vi "更新列首行首.vi"(0 "MulticolumnListbox输入":refnum<vi>, 1 "Coords":T1, 3 "列首？":bool=TRUE, 4 "行首？":bool=TRUE, 5 "项名？":bool=TRUE, 7 "编辑单元格":bool=TRUE) -> (13 "边界内？":bool, 14 "列首":string[](array[string]), 16 "行首":string[](array[string]), 18 "项名":string[][](array[string]), 19 "错误输出":errorcluster)   [LabVIEW 2016]
uses:
  <vilib>/Utility/miscctls.llb/LVPoint32TypeDef.ctl
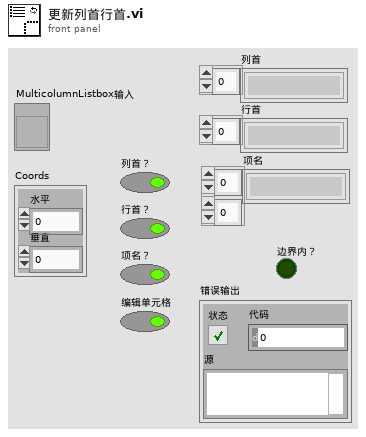
[diagram p1: front panel]
types:
  T1 = typedef "LVPoint32TypeDef.ctl" = cluster{"Horizontal":i32, "Vertical":i32}
  T2 = typedef "LVRowAndColumnTypeDef.ctl" = cluster{"Row":i32, "Column":i32}
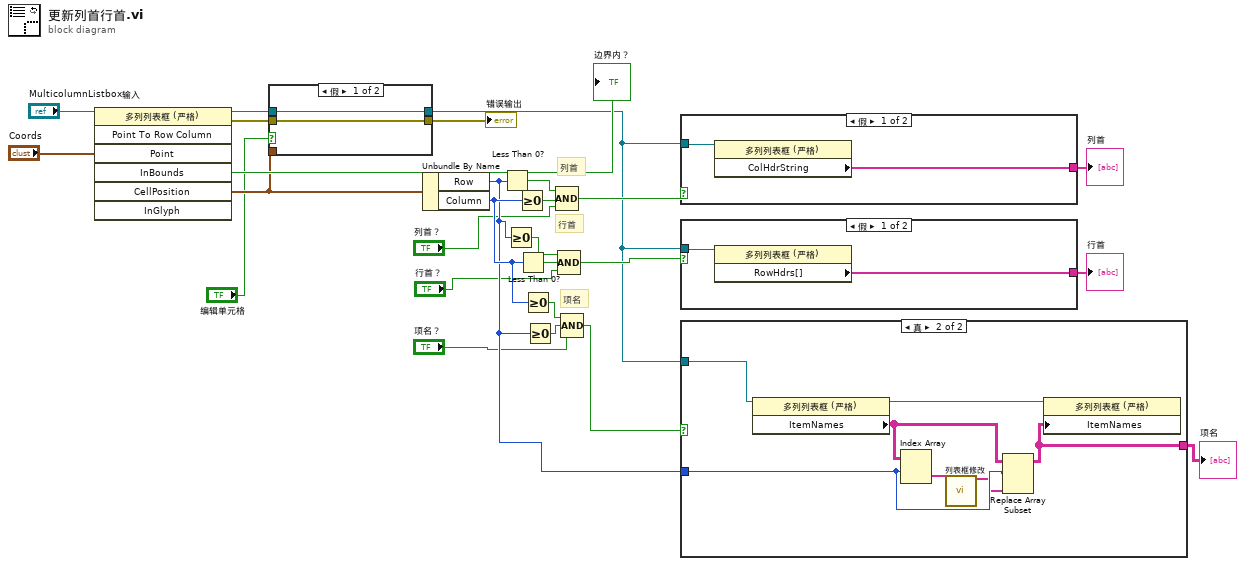
[diagram p0: block diagram]
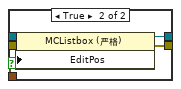
[diagram p2: hidden frame]
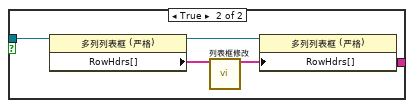
[diagram p3: hidden frame]
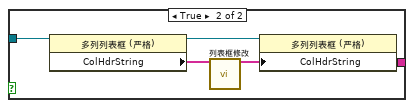
[diagram p4: hidden frame]
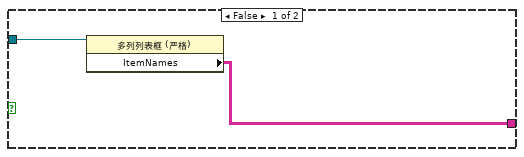
[diagram p5: hidden frame]
diagram:
  # "项名"
  # "列首"
  # "行首"
  n1 = invoke class="多列列表框 (严格)" method="Point To Row Column"(reference="MulticolumnListbox输入", "Point"="Coords") -> (reference out=w6:refnum<vi>, error out=w4:errorcluster, "InBounds"=→"边界内？":bool, "CellPosition"=w2:T2)  [unwired: 5 in, 3 out]
  n2 = case shown="假" "编辑单元格" {
    tunnel: w6 -> [w28 w33]
    tunnel: [w28 w32] -> w5
    tunnel: w4 -> [w27 w31]
    tunnel: [w27 w30] -> w3
    tunnel: w2 -> [_ w29]
    frame False {
    }
    frame True {
      n3 = property class="MCListbox (严格)"(reference=w33, error in=w31, "EditPos"=w29) -> (reference out=w32:refnum<vi>, error out=w30:errorcluster)
    }
  }
  "错误输出" <- w3
  n4 = Unbundle By Name(w2) -> ("Row"=w13:i32, "Column"=w14:i32)
  n5 = Less Than 0?(x=w13) -> (x < 0?=w23:bool)
  n6 = Greater Or Equal To 0?(x=w13) -> (x >= 0?=w22:bool)
  n7 = Greater Or Equal To 0?(x=w14) -> (x >= 0?=w24:bool)
  n8 = Less Than 0?(x=w14) -> (x < 0?=w21:bool)
  n9 = Greater Or Equal To 0?(x=w14) -> (x >= 0?=w12:bool)
  n10 = Greater Or Equal To 0?(x=w13) -> (x >= 0?=w11:bool)
  n11 = Compound Arithmetic op=AND ("复合运算")(w23, w24, "列首？") -> (w19:bool)
  n12 = Compound Arithmetic op=AND ("复合运算")(w22, w21, "行首？") -> (w18:bool)
  n13 = Compound Arithmetic op=AND ("复合运算")(w12, w11, "项名？") -> (w10:bool)
  n14 = case shown="假" w19 {
    tunnel: w5 -> [w35 w37]
    tunnel: [w34 w36] -> w17
    frame False {
      n15 = property class="多列列表框 (严格)"(reference=w35) -> ("ColHdrString"=w34:string[])  [unwired: 1 in, 2 out]
    }
    frame True {
      n16 = property class="多列列表框 (严格)"(reference=w37) -> (reference out=w38:refnum<vi>, "ColHdrString"=w39:string[])  [unwired: 1 in, 1 out]
      n17 = call "列表框修改.vi"("输入/修改"=w39) -> ("增加测试信息"=w36:string[])  [unwired: 13 in, 1 out]
      n18 = property class="多列列表框 (严格)"(reference=w38, "ColHdrString"=w36) -> ()  [unwired: 1 in, 2 out]
    }
  }
  "列首" <- w17
  n19 = case shown="假" w18 {
    tunnel: w5 -> [w41 w43]
    tunnel: [w40 w42] -> w16
    frame False {
      n20 = property class="多列列表框 (严格)"(reference=w41) -> ("RowHdrs[]"=w40:string[])  [unwired: 1 in, 2 out]
    }
    frame True {
      n21 = property class="多列列表框 (严格)"(reference=w43) -> (reference out=w44:refnum<vi>, "RowHdrs[]"=w45:string[])  [unwired: 1 in, 1 out]
      n22 = call "列表框修改.vi"("输入/修改"=w45) -> ("增加测试信息"=w42:string[])  [unwired: 13 in, 1 out]
      n23 = property class="多列列表框 (严格)"(reference=w44, "RowHdrs[]"=w42) -> ()  [unwired: 1 in, 2 out]
    }
  }
  "行首" <- w16
  n24 = case shown="真" w10 {
    tunnel: w13 -> [_ w51]
    tunnel: w5 -> [w47 w53]
    tunnel: [w46 w48] -> w15
    frame False {
      n25 = property class="多列列表框 (严格)"(reference=w47) -> ("ItemNames"=w46:string[][])  [unwired: 1 in, 2 out]
    }
    frame True {
      n26 = property class="多列列表框 (严格)"(reference=w53) -> (reference out=w54:refnum<vi>, "ItemNames"=w52:string[][])  [unwired: 1 in, 1 out]
      n27 = Index Array(array=w52, index (row)=w51) -> (element=w50:string[])  [unwired: 1 in]
      n28 = call "列表框修改.vi"("输入/修改"=w50) -> ("增加测试信息"=w49:string[])  [unwired: 13 in, 1 out]
      n29 = Replace Array Subset(array=w52, new element=w49, index (row)=w51) -> (w48:string[][])  [unwired: 1 in]
      n30 = property class="多列列表框 (严格)"(reference=w54, "ItemNames"=w48) -> ()  [unwired: 1 in, 2 out]
    }
  }
  "项名" <- w15
